vi "Read RS-xxx To GPIB ConvBox Data Structure.vi"(8 "error in (no error)":errorcluster, 11 "Listener in":refnum<class "Listener.lvclass">) -> (0 "error out":errorcluster, 2 "RS-xxx To GPIB ConvBox Data Structure":T1, 3 "Listener out":refnum<class "Listener.lvclass">)   [LabVIEW 2019, in "Listener.lvclass"]
uses:
  Listener.lvclass
  ListenerClassControls/RS-xxx To GPIB ConvBox Data Structure.ctl
  Listener.lvclass/Listener.ctl
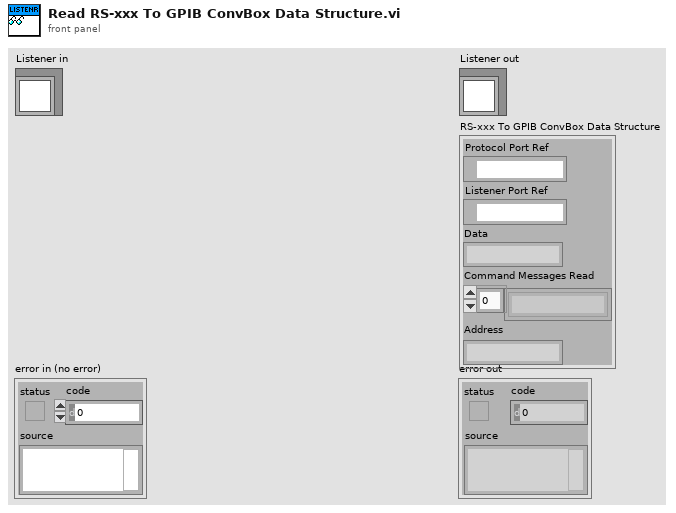
[diagram p1: front panel]
types:
  T1 = typedef "Listener.lvclass/RS-xxx To GPIB ConvBox Data Structure.ctl" = cluster{"Protocol Port Ref":refnum<visa-resource-name>, "Listener Port Ref":refnum<visa-resource-name>, "Data":string, "Command Messages Read":string[], "Address":string}
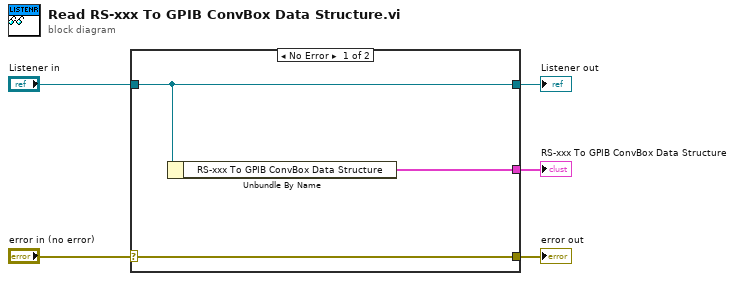
[diagram p0: block diagram]
diagram:
  n1 = case shown="No Error" "error in (no error)" {
    selector: "error in (no error)" -> [w8 w9]
    tunnel: [w8 w9] -> w4
    tunnel: [w7 w10] -> w2
    tunnel: "Listener in" -> [w7 w10]
    tunnel: [w6 _] -> w1
    frame No Error {
      n2 = Unbundle By Name(w7) -> ("RS-xxx To GPIB ConvBox Data Structure"=w6:T1)
    }
    frame Error {
    }
  }
  "error out" <- w4
  "Listener out" <- w2
  "RS-xxx To GPIB ConvBox Data Structure" <- w1
